vi "BRig_Host_dataRunState_dataPlot_reward2.vi"() -> (2 "output_idx_dataPlot_reward2":i32)   [LabVIEW 2014]
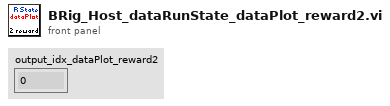
[diagram p1: front panel]
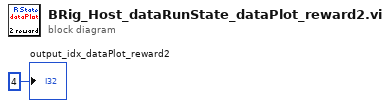
[diagram p0: block diagram]
diagram:
  "output_idx_dataPlot_reward2" <- 4 ("output_idx_dataTS")
